vi "Test DVR Flatten.vi"() -> ()   [LabVIEW 2021]
uses:
  CIFfifo.lvclass
  CIFfifo.lvclass/CIFfifo.ctl
  Utilities/Flatten Header.vi
  Flatten/DVR Flatten.vi/6fdbece9-bad6-4a8e-9bf7-fe1528478dd6.vi
  Accessors/Write Payload Length.vi
  Accessors/Read Header.vi
  Utilities/Unflatten Header.vi
  CIFCore/Common/Utilities/Add Error.vi
  Flatten/DVR Flatten.vi/6fdbece9-bad6-4a8e-9bf7-fe1528478dd6.vi/c28b0ead-42ad-4072-80a2-aca7f2bd7ce3.vi
  CIFCore/Common/Utilities/Append Error Location.vi
panel:
  out "Array":i32[](array[numeric])
  out "Data out":u64[](array[numeric])
  out "error out":errorcluster
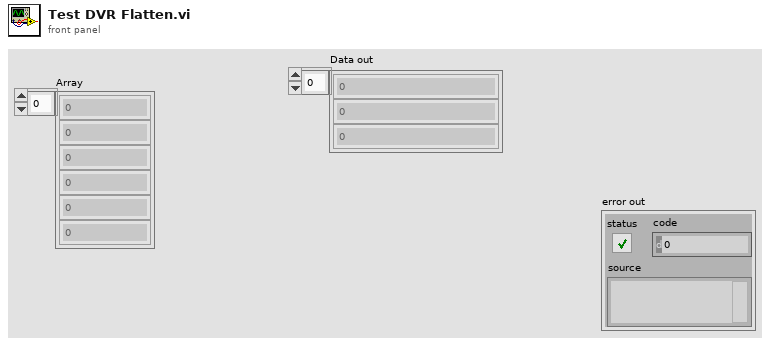
[diagram p1: front panel]
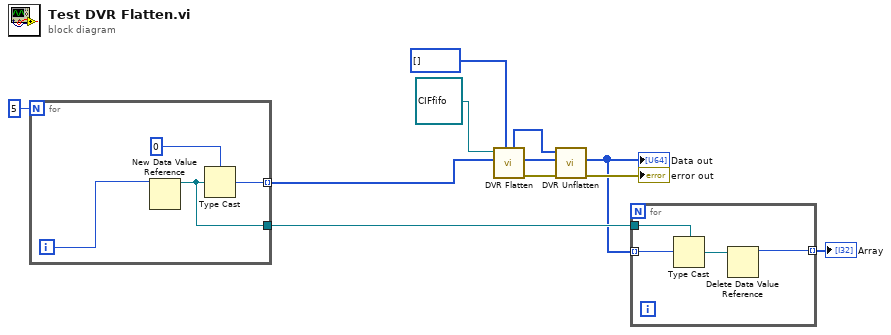
[diagram p0: block diagram]
diagram:
  n1 = for {
    N: 5 -> [_]
    tunnel: [w13] -> w4 mode=indexing
    tunnel: [w12] -> w3
    i -> [w14]
    n2 = New Data Value Reference(data value=w14) -> (data value reference=w12:refnum<data-value>)  [unwired: 1 in, 1 out]
    n3 = Type Cast(type=u64 0 ("unsigned 64bit integer"), x=w12) -> (*(type *) &x=w13:u64)
  }
  n4 = call "DVR Flatten.vi"("payload in"=u8[] [], "Data In"=w4, "CIFFifo in"=refnum<class "CIFfifo.lvclass"> refnum) -> ("error out"=w11:errorcluster, "Data out"=w6:u64[], "payload out"=w10:u8[])  [unwired: 4 in, 2 out]
  n5 = call "DVR Unflatten.vi"("error in (no error)"=w11, "Data In"=w6, "Flatten Data in"=w10) -> ("error out"=→"error out":errorcluster, "Data out"=w1:u64[])  [unwired: 5 in, 2 out]
  "Data out" <- w1
  n6 = for {
    tunnel: w1 -> [w19] mode=indexing
    tunnel: w3 -> [w17]
    tunnel: [w16] -> w2 mode=indexing
    n7 = Type Cast(type=w17, x=w19) -> (*(type *) &x=w18:refnum<data-value>)
    n8 = Delete Data Value Reference(data value reference=w18) -> (data value=w16:i32)  [unwired: 1 in, 1 out]
  }
  "Array" <- w2
